vi "Example_TronVIEWGame.vi"() -> ()   [LabVIEW 2015]
uses:
  TronviewGame/Game/GameResult.ctl
  TronviewGame/Board/BoardSize.ctl
  TronviewGame/Game/Game.lvclass/Game.ctl
  TronviewGame/Board/Board.lvclass
  TronviewGame/Game/Game.lvclass
  TronviewGame/Player/Player.lvclass
  TronviewGame/TronviewGame.lvlib
panel:
  out "Array 2":u32[][](array[colorbox])
  out "GameResult":T1
  out "Finished?":bool
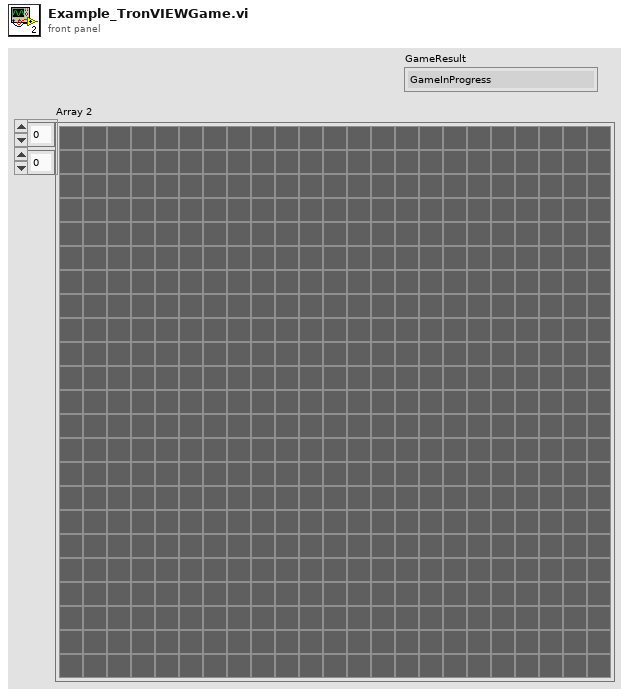
[diagram p1: front panel]
types:
  T1 = typedef "TronviewGame.lvlib/Game.lvclass/GameResult.ctl" = enum16{"GameInProgress", "Draw", "Player1Won", "Player2Won"}
  T2 = typedef "TronviewGame.lvlib/Board.lvclass/BoardSize.ctl" = cluster{"Columns":u32, "Rows":u32}
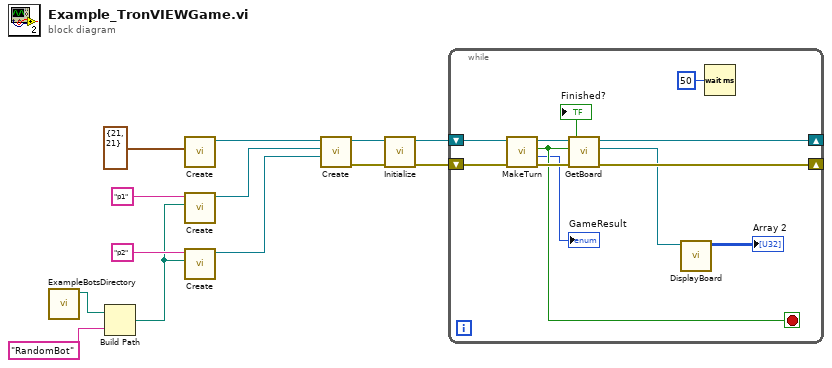
[diagram p0: block diagram]
diagram:
  n1 = call "ExampleBotsDirectory.vi"() -> ("stripped path"=w3:path)  [unwired: 11 in]
  n2 = Build Path(base path=w3, name or relative path="RandomBot") -> (appended path=w1:path)
  n3 = call "Create.vi"("Size"=T2 {"Columns"=21, "Rows"=21}) -> ("Board out"=w12:refnum<class "Board.lvclass">)  [unwired: 9 in, 1 out]
  n4 = call "Create.vi"("PlayerFolder"=w1, "PlayerName"="p1") -> ("Player out"=w7:refnum<class "Player.lvclass">)  [unwired: 8 in, 1 out]
  n5 = call "Create.vi"("PlayerFolder"=w1, "PlayerName"="p2") -> ("Player out"=w6:refnum<class "Player.lvclass">)  [unwired: 8 in, 1 out]
  n6 = call "Create.vi"("Player2"=w6, "Player1"=w7, "Board"=w12) -> ("error out"=w10:errorcluster, "Game out"=w11:refnum<class "Game.lvclass">)  [unwired: 7 in]
  n7 = call "Initialize.vi"("error in (no error)"=w10, "Game in"=w11) -> ("error out"=w8:errorcluster, "Game out"=w9:refnum<class "Game.lvclass">)  [unwired: 8 in]
  n8 = while {
    shift-right: [w20] -> _
    shift-left: w9 -> [w24]
    shift-right: [w19] -> _
    shift-left: w8 -> [w23]
    stop <- w17 stop-if-true
    n9 = call "MakeTurn.vi"("error in (no error)"=w23, "Game in"=w24) -> ("error out"=w21:errorcluster, "GameResult"=→"GameResult":T1, "Finished?"=w17:bool, "Game out"=w22:refnum<class "Game.lvclass">)  [unwired: 6 in]
    "Finished?" <- w17
    n10 = call "GetBoard.vi"("error in (no error)"=w21, "Game in"=w22) -> ("error out"=w19:errorcluster, "TronviewGame.lvlib:Board.lvclass"=w15:refnum<class "Board.lvclass">, "Game out"=w20:refnum<class "Game.lvclass">)  [unwired: 7 in]
    n11 = call "DisplayBoard.vi"("Board"=w15) -> ("Array"=→"Array 2":u32[][])  [unwired: 10 in]
    n12 = Wait (ms)(milliseconds to wait=u32 50) -> ()  [unwired: 1 out]
  }
